vi "测量.vi"(8 "错误输入（无错误）":errorcluster, 10 "测量队列":T1(array[cluster]), 11 "VISA资源名称":refnum<visa-resource-name>) -> (0 "错误输出":errorcluster, 2 "数组":dbl[](array[numeric]), 3 "VISA资源名称输出":refnum<visa-resource-name>)   [LabVIEW 2020]
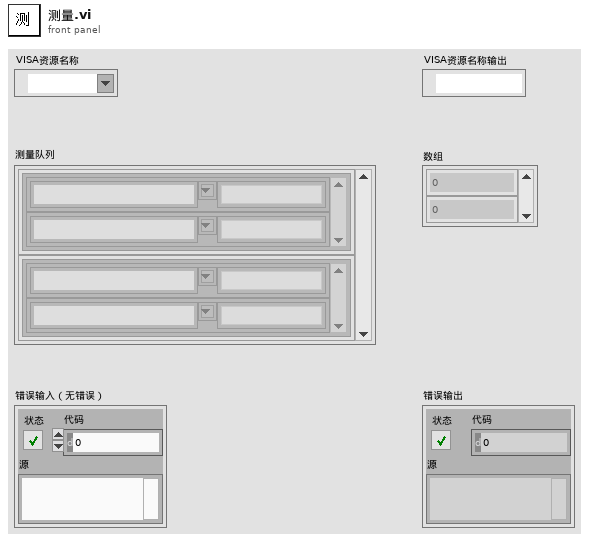
[diagram p1: front panel]
types:
  T1 = cluster{"测量参数":cluster{"设置项":string, "值":string}[]}[]
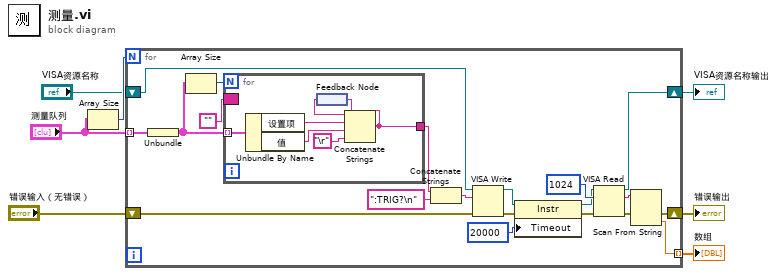
[diagram p0: block diagram]
diagram:
  n1 = Array Size(array="测量队列") -> (size(s)=w6:i32)
  n2 = for {
    N: w6 -> [_]
    tunnel: "测量队列" -> [w27] mode=indexing
    tunnel: [w19] -> w1 mode=indexing
    shift-right: [w14] -> w2
    shift-left: "VISA资源名称" -> [w20]
    shift-right: [w8] -> w3
    shift-left: "错误输入（无错误）" -> [w21]
    n3 = Unbundle(w27) -> ("测量参数"=w25:cluster{"设置项":string, "值":string}[])
    n4 = Array Size(array=w25) -> (size(s)=w26:i32)
    n5 = for {
      N: w26 -> [_]
      tunnel: w25 -> [w33] mode=indexing
      tunnel: [w28] -> w24
      border: "" -> [_]
      n6 = Unbundle By Name(w33) -> ("设置项"=w32:string, "值"=w31:string)
      n7 = feedback #1() -> (w29:string)
      n8 = Concatenate Strings(w29, w32, w31, "\r") -> (w28:string)
      n9 = feedback-in #1(w28) -> ()
    }
    n10 = Concatenate Strings(w24, ":TRIG?\n" ("字符串")) -> (w22:string)
    n11 = VISA Write(VISA resource name=w20, write buffer=w22, error in (no error)=w21) -> (VISA resource name out=w12:refnum<visa-resource-name>, error out=w13:errorcluster)  [unwired: 1 out]
    n12 = property class="Instr"(reference=w12, error in=w13, "Timeout"=u32 20000 ("General Settings:Timeout Value")) -> (reference out=w11:refnum<visa-resource-name>, error out=w10:errorcluster)
    n13 = VISA Read(VISA resource name=w11, byte count=u32 1024 ("字节总数"), error in (no error)=w10) -> (VISA resource name out=w14:refnum<visa-resource-name>, read buffer=w15:string, error out=w16:errorcluster)  [unwired: 1 out]
    n14 = Scan From String(input string=w15, error in=w16) -> (error out=w8:errorcluster, output 1=w19:dbl)  [unwired: 3 in, 2 out]
  }
  "错误输出" <- w3
  "VISA资源名称输出" <- w2
  "数组" <- w1
